vi "Launch Models.vi"(10 "Top Level Path":path, 11 "Message Enqueuer in":refnum<class "Message Enqueuer.lvclass">) -> (3 "Message Enqueuer out":refnum<class "Message Enqueuer.lvclass">)   [LabVIEW 2013]
uses:
  <vilib>/ActorFramework/Message Enqueuer/Message Enqueuer.lvclass
  <vilib>/ActorFramework/Actor/Actor.lvclass
  Models/Main Model/Main Model.lvclass
  Models/Project Model/Project Model.lvclass
  Models/Create Project Model/Create Project Model.lvclass
  Models/Edit Project Model/Edit Project Model.lvclass
  Models/Sensor Model/Sensor Model.lvclass
  Models/Create Sensor Model/Create Sensor Model.lvclass
  Models/Edit Sensor Model/Edit Sensor Model.lvclass
  Models/Test Node Model/Test Node Model.lvclass
  Models/Create Test Node Model/Create Test Node Model.lvclass
  Models/Edit Test Node Model/Edit Test Node Model.lvclass
  Models/Test Channel Model/Test Channel Model.lvclass
  Models/Create Test Channel Model/Create Test Channel Model.lvclass
  Models/Edit Test Channel Model/Edit Test Channel Model.lvclass
  Models/HVAC System Model/HVAC System Model.lvclass
  Models/Hot And Cold Source Unit Model/Hot And Cold Source Unit Model.lvclass
  <vilib>/ActorFrameworkMVC/UI Controller Messages/Launch Model Actor Msg/Launch Model Actor Msg.lvclass/Launch Model Actor Msg.ctl
  <vilib>/ActorFramework/Message Enqueuer/Message Enqueuer.lvclass/Message Enqueuer.ctl
  Models/Abstract Model Messages/Set Top Level Path Msg/Set Top Level Path Msg.lvclass/Set Top Level Path Msg.ctl
  <vilib>/ActorFramework/Message Enqueuer/Enqueue.vi
  <vilib>/ActorFramework/Message Priority Queue/Priority Enqueue.vi
  <vilib>/ActorFrameworkMVC/UI Controller Messages/Launch Model Actor Msg/Launch Model Actor Msg.lvclass
  Models/Abstract Model Messages/Set Top Level Path Msg/Set Top Level Path Msg.lvclass
  <vilib>/ActorFrameworkMVC/UI Controller Messages/Get Model Actor Enqueuer Msg/Get Model Actor Enqueuer Msg.lvclass
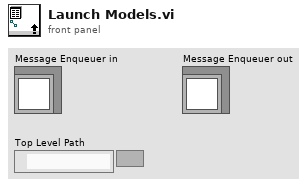
[diagram p1: front panel]
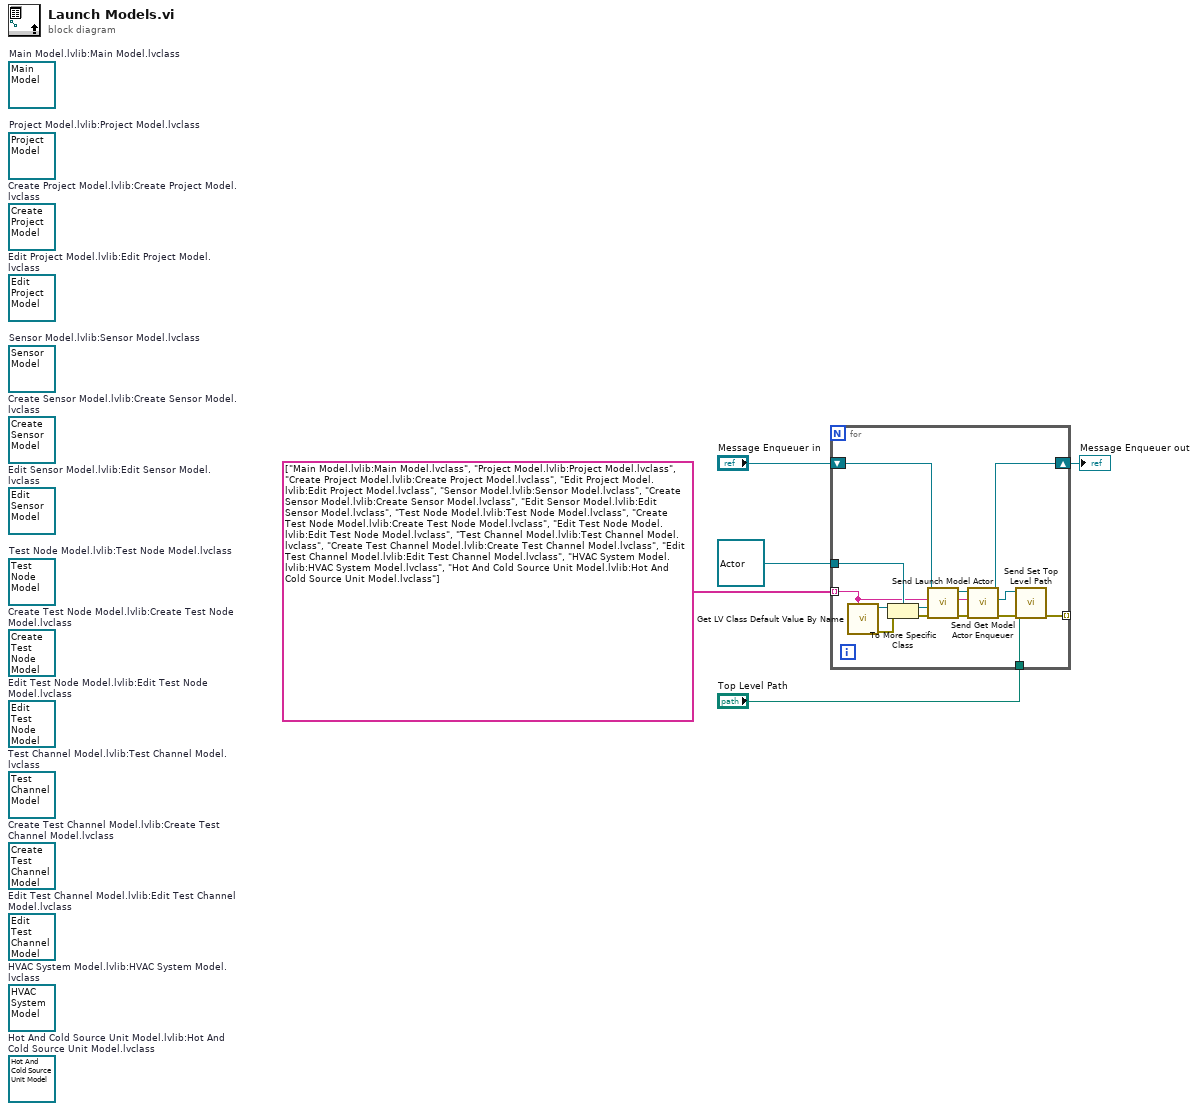
[diagram p0: block diagram]
diagram:
  (unwired) refnum<class "Hot And Cold Source Unit Model.lvclass"> refnum  # Hot And Cold Source Unit Model.lvlib:Hot And Cold Source Unit Model.lvclass
  (unwired) refnum<class "HVAC System Model.lvclass"> refnum  # HVAC System Model.lvlib:HVAC System Model.lvclass
  (unwired) refnum<class "Edit Test Channel Model.lvclass"> refnum  # Edit Test Channel Model.lvlib:Edit Test Channel Model.lvclass
  (unwired) refnum<class "Create Test Channel Model.lvclass"> refnum  # Create Test Channel Model.lvlib:Create Test Channel Model.lvclass
  (unwired) refnum<class "Test Channel Model.lvclass"> refnum  # Test Channel Model.lvlib:Test Channel Model.lvclass
  (unwired) refnum<class "Edit Test Node Model.lvclass"> refnum  # Edit Test Node Model.lvlib:Edit Test Node Model.lvclass
  (unwired) refnum<class "Create Test Node Model.lvclass"> refnum  # Create Test Node Model.lvlib:Create Test Node Model.lvclass
  (unwired) refnum<class "Test Node Model.lvclass"> refnum  # Test Node Model.lvlib:Test Node Model.lvclass
  (unwired) refnum<class "Edit Sensor Model.lvclass"> refnum  # Edit Sensor Model.lvlib:Edit Sensor Model.lvclass
  (unwired) refnum<class "Create Sensor Model.lvclass"> refnum  # Create Sensor Model.lvlib:Create Sensor Model.lvclass
  (unwired) refnum<class "Sensor Model.lvclass"> refnum  # Sensor Model.lvlib:Sensor Model.lvclass
  (unwired) refnum<class "Edit Project Model.lvclass"> refnum  # Edit Project Model.lvlib:Edit Project Model.lvclass
  (unwired) refnum<class "Create Project Model.lvclass"> refnum  # Create Project Model.lvlib:Create Project Model.lvclass
  (unwired) refnum<class "Project Model.lvclass"> refnum  # Project Model.lvlib:Project Model.lvclass
  (unwired) refnum<class "Main Model.lvclass"> refnum  # Main Model.lvlib:Main Model.lvclass
  n1 = for {
    shift-right: [w11] -> w4
    shift-left: "Message Enqueuer in" -> [w16]
    tunnel: refnum<class "Actor.lvclass"> refnum ("UI Actor") -> [w19]
    tunnel: string[] ["Main Model.lvlib:Main Model.lvclass", "Project Model.lvlib:Project Model.lvclass", "Create Project Model.lvlib:Create Project Model.lvclass", "Edit Project Model.lvlib:Edit Project Model.lvclass", "Sensor Model.lvlib:Sensor Model.lvclass", "Create Sensor Model.lvlib:Create Sensor Model.lvclass", "Edit Sensor Model.lvlib:Edit Sensor Model.lvclass", "Test Node Model.lvlib:Test Node Model.lvclass", "Create Test Node Model.lvlib:Create Test Node Model.lvclass", "Edit Test Node Model.lvlib:Edit Test Node Model.lvclass", "Test Channel Model.lvlib:Test Channel Model.lvclass", "Create Test Channel Model.lvlib:Create Test Channel Model.lvclass", "Edit Test Channel Model.lvlib:Edit Test Channel Model.lvclass", "HVAC System Model.lvlib:HVAC System Model.lvclass", "Hot And Cold Source Unit Model.lvlib:Hot And Cold Source Unit Model.lvclass"] -> [w14] mode=indexing
    tunnel: "Top Level Path" -> [w12]
    tunnel: [w6] -> _ mode=indexing
    n2 = call <vilib>:"Get LV Class Default Value By Name.vi"("class name"=w14) -> ("error out"=w7:errorcluster, "object"=w18:refnum<class>)  [unwired: 9 in]
    n3 = To More Specific Class(target class=w19, reference=w18, error in=w7) -> (specific class reference=w17:refnum<class "Actor.lvclass">, error out=w8:errorcluster)
    n4 = call <vilib>:"Send Launch Model Actor.vi"("error in (no error)"=w8, "Model Actor"=w17, "Model Name"=w14, "Message Enqueuer"=w16) -> ("error out"=w9:errorcluster, "Message Enqueuer out"=w15:refnum<class "Message Enqueuer.lvclass">)  [unwired: 6 in]
    n5 = call <vilib>:"Send Get Model Actor Enqueuer.vi"("error in (no error)"=w9, "Model Name"=w14, "Message Enqueuer in"=w15) -> ("error out"=w10:errorcluster, "Reply"=w13:refnum<class "Message Enqueuer.lvclass">, "Message Enqueuer out"=w11:refnum<class "Message Enqueuer.lvclass">)  [unwired: 5 in, 1 out]
    n6 = call "Send Set Top Level Path.vi"("error in (no error)"=w10, "Top Level Path"=w12, "Message Enqueuer"=w13) -> ("error out"=w6:errorcluster)  [unwired: 7 in, 1 out]
  }
  "Message Enqueuer out" <- w4
